vi "Wait for Specific Response.vi"(0 "TCP Connection In":refnum<k5>, 1 "Next response (t)":bool=TRUE, 5 "Expected Type":T3=enum."NONE", 7 "Expected Subtype (none)":T1, 9 "Expected Message Start (\"\":any)":string, 11 "error in":errorcluster, 12 "Timeout (250 ms)":i32=250) -> (4 "TCP Connection Out":refnum<k5>, 6 "TCP Messages":string[](array[string]), 8 "Desired Response":T2, 15 "error out":errorcluster)   [LabVIEW 2011, in "ART2 Test Panel.lvlib"]
doc: "If 'next response' is false, then the VI will ignore responses that do not match the response, waiting for a match. If no match is found by the timeout time, the VI returns an error."
uses:
  ART2 Test Panel.lvlib
  Controls/NART TCP Response Types.ctl
  Controls/NART Message.ctl
  Controls/NART Response Subtype.ctl
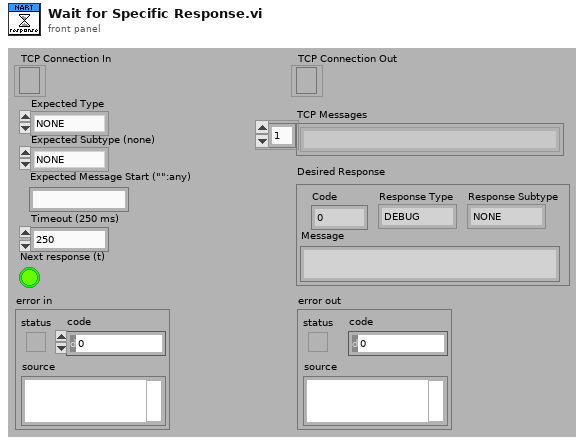
[diagram p1: front panel]
types:
  T1 = typedef "ART2 Test Panel.lvlib/NART Response Subtype.ctl" = enum16{"NONE", "OK", "ON", "OFF", "BEGIN", "DONE"}
  T2 = typedef "ART2 Test Panel.lvlib/NART Message.ctl" = cluster{"Code":dbl, "Response Type":T3, "Response Subtype":T1, "Message":string}
  T3 = typedef "ART2 Test Panel.lvlib/NART TCP Response Types.ctl" = enum16{"DEBUG", "CONTROL", "INFO", "WARNING", "ERROR", "NONE"}
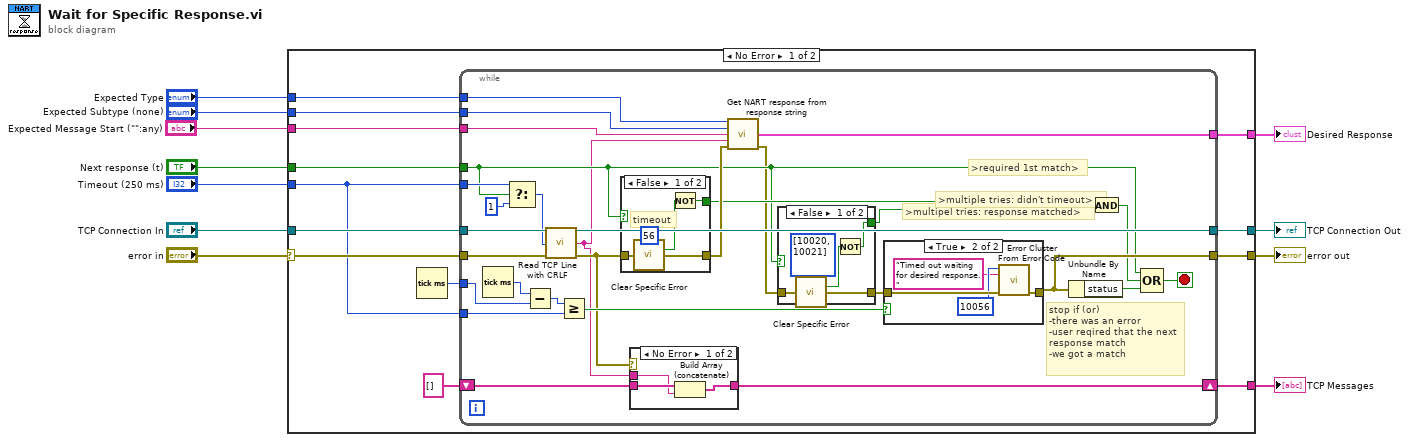
[diagram p0: block diagram]
diagram:
  n1 = case shown="No Error" "error in" {
    selector: "error in" -> [w24 w76]
    tunnel: [w15 w76] -> w8
    tunnel: "TCP Connection In" -> [w23 w75]
    tunnel: [w22 w75] -> w10
    tunnel: "Timeout (250 ms)" -> [w16 _]
    tunnel: [w19 _] -> w6
    tunnel: "Expected Type" -> [w21 _]
    tunnel: "Expected Subtype (none)" -> [w20 _]
    tunnel: "Next response (t)" -> [w18 _]
    tunnel: [w14 _] -> w2
    tunnel: "Expected Message Start (\"\":any)" -> [w12 _]
    frame No Error {
      n2 = Tick Count (ms)() -> (millisecond timer value=w17:u32)
      n3 = while {
        tunnel: w24 -> [w53]
        tunnel: w23 -> [w52]
        tunnel: [w51] -> w22
        tunnel: w21 -> [w50]
        tunnel: w20 -> [w49]
        tunnel: [w31] -> w19
        tunnel: w16 -> [w34]
        tunnel: w18 -> [w33]
        tunnel: w17 -> [w46]
        tunnel: w16 -> [w44]
        tunnel: [w39] -> w15
        shift-right: [w30] -> w14
        shift-left: string[] [] -> [w29]
        tunnel: w12 -> [w25]
        stop <- w40 stop-if-true
        # ">required 1st match>"
        # ">multipel tries: response matched>"
        # ">multiple tries: didn't timeout>"
        # "stop if (or)\n-there was an error\n-user reqired that the next response match\n-we got a match"
        n4 = Tick Count (ms)() -> (millisecond timer value=w47:u32)
        n5 = Select(t=w34, s=w33, f=1) -> (s? t:f=w48:i32)
        n6 = Subtract(x=w47, y=w46) -> (x-y=w45:u32)
        n7 = call "Read TCP Line with CRLF.vi"("TCP Connection In"=w52, "timeout ms (100)"=w48, "error in"=w53) -> ("TCP Connection Out"=w51:refnum<k5>, "TCP Line"=w26:string, "error out"=w27:errorcluster)  [unwired: 10 in]
        n8 = Greater Or Equal?(x=w45, y=w44) -> (x >= y?=w43:bool)
        n9 = case shown="False" w33 {
          tunnel: w27 -> [w68 w69]
          tunnel: [w67 w69] -> w42
          tunnel: [w64 _] -> w37
          frame False {
            # "timeout"
            n10 = call "Clear Specific Error.vi"("Specific Error Number (0: none)"=56 ("Specific Error Number"), "error in"=w68) -> ("Error Cleared?"=w65:bool, "error out"=w67:errorcluster)  [unwired: 12 in]
            n11 = Not(x=w65) -> (.not. x?=w64:bool)
          }
          frame True {
            # "1 try"
          }
        }
        n12 = case shown="No Error" w27 {
          tunnel: [w56 w57] -> w30
          tunnel: w29 -> [w55 w57]
          tunnel: w26 -> [w54 _]
          frame No Error {
            n13 = Build Array (concatenate)(w55, w54) -> (w56:string[])
          }
          frame Error {
          }
        }
        n14 = call "Get NART response from response string.vi"("Expected Response"=w50, "Response Subtype"=w49, "Expected Message start (\"\":any)"=w25, "TCP Line"=w26, "error in (no error)"=w42) -> ("NART Message"=w31:T2, "error out"=w28:errorcluster)  [unwired: 9 in]
        n15 = case shown="False" w33 {
          tunnel: w28 -> [w62 w63]
          tunnel: [w61 w63] -> w38
          tunnel: [w59 _] -> w36
          frame False {
            n16 = call "Clear Specific Error.vi"("Error Numbers Array (emtpy)"=i32[] [10020, 10021] ("Error Numbers Array"), "error in"=w62) -> ("Error Cleared?"=w60:bool, "error out"=w61:errorcluster)  [unwired: 12 in]
            n17 = Not(x=w60) -> (.not. x?=w59:bool)
          }
          frame True {
            # "1 try"
          }
        }
        n18 = case shown="True" w43 {
          tunnel: w38 -> [w70 w74]
          tunnel: [w70 w72] -> w39
          frame False {
          }
          frame True {
            n19 = call <vilib>:"Error Cluster From Error Code.vi"("error in (no error)"=w74, "error message (\"\")"="Timed out waiting for desired response." ("format string"), "error code (0)"=10056) -> ("error out"=w72:errorcluster)  [unwired: 6 in]
          }
        }
        n20 = Unbundle By Name(w39) -> ("status"=w41:bool)
        n21 = And(x=w37, y=w36) -> (x .and. y?=w35:bool)
        n22 = Compound Arithmetic op=OR(w33, w35, w41) -> (w40:bool)
      }
    }
    frame Error {
    }
  }
  "TCP Connection Out" <- w10
  "error out" <- w8
  "Desired Response" <- w6
  "TCP Messages" <- w2
